vi "sendValveSignal-v02.2.vi"(0 "daq_do":tag="Dev1/ai0:1", 3 "Valve1?":bool, 5 "ChangeToValve":u16, 9 "CurrentValve":u16, 11 "controls array in":refnum<vi>[](array[refnum]), 12 "Set Status":bool, 13 "error in":errorcluster) -> (6 "ValveSetTo":u16, 10 "valve changed?":bool, 14 "error out":errorcluster, 15 "control array out":refnum<vi>[](array[refnum]))   [LabVIEW 2019]
uses:
  <vilib>/DAQmx/write.llb/DAQmx Write (Digital 1D Bool NChan 1Samp 1Line).vi
  <vilib>/DAQmx/miscellaneous.llb/DAQmx Fill In Error Info.vi
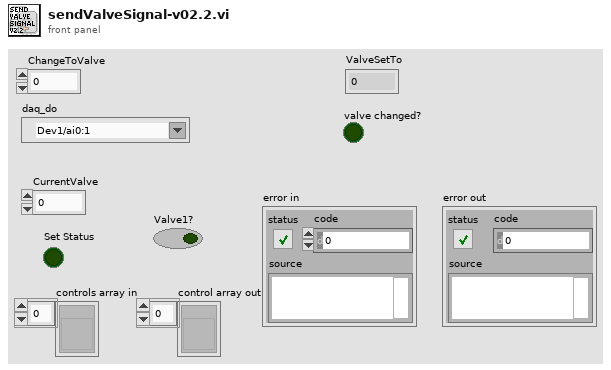
[diagram p1: front panel]
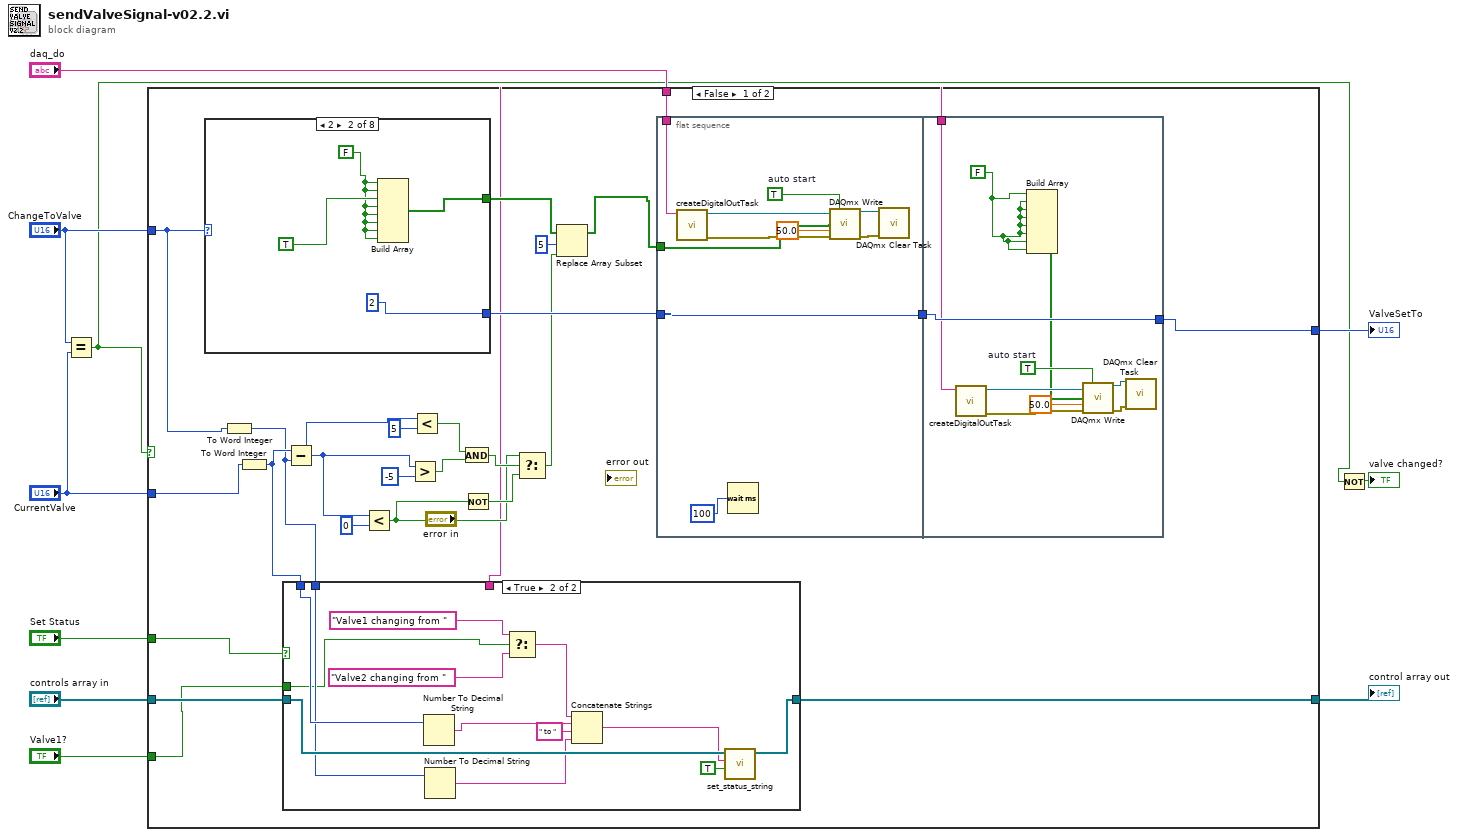
[diagram p0: block diagram]
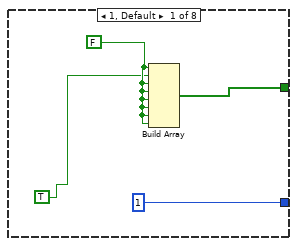
[diagram p3: hidden frame]
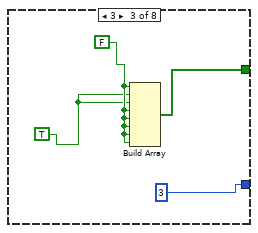
[diagram p4: hidden frame]
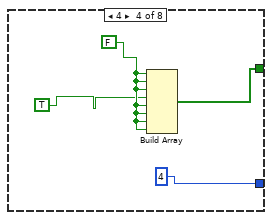
[diagram p5: hidden frame]
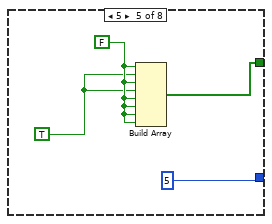
[diagram p6: hidden frame]
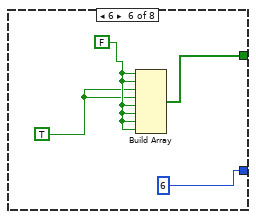
[diagram p7: hidden frame]
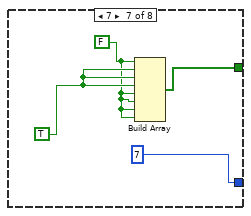
[diagram p8: hidden frame]
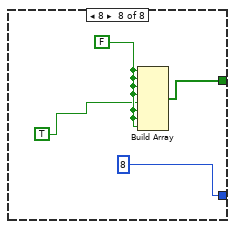
[diagram p9: hidden frame]
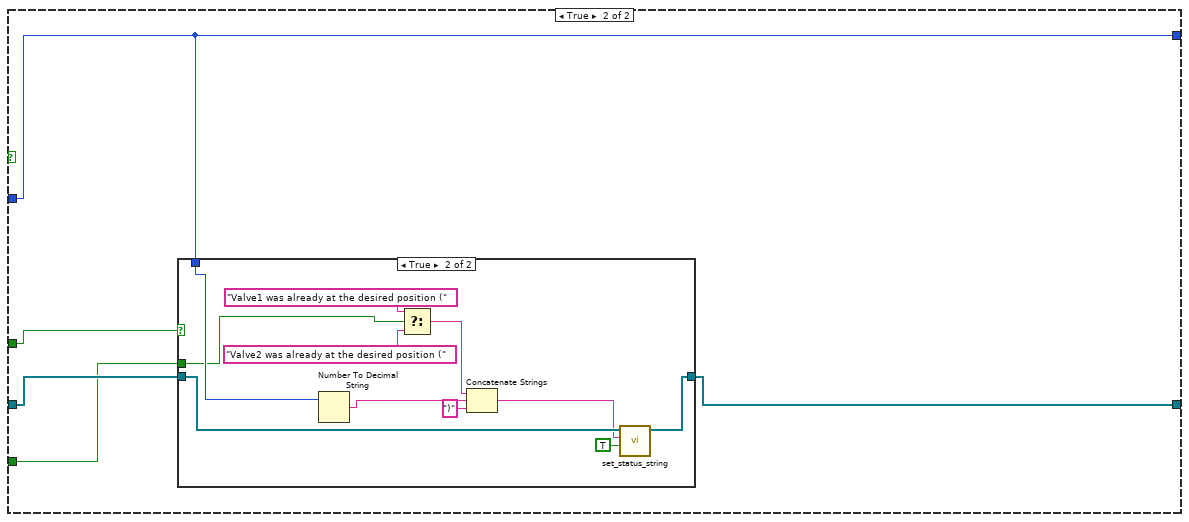
[diagram p10: hidden frame]
diagram:
  n1 = Equal?(x="ChangeToValve", y="CurrentValve") -> (x = y?=w1:bool)
  n2 = case shown="False" w1 {
    tunnel: [w33 w103] -> w10
    tunnel: "Set Status" -> [w19 w106]
    tunnel: "controls array in" -> [w18 w105]
    tunnel: [w17 w102] -> w7
    tunnel: "daq_do" -> [w16 _]
    tunnel: "Valve1?" -> [w13 w104]
    tunnel: "ChangeToValve" -> [w12 _]
    tunnel: "CurrentValve" -> [w11 w103]
    frame False {
      n3 = case shown="2" w12 {
        tunnel: [w73 w77 w81 w85 w89 w93 w97 w101] -> w23
        tunnel: [u16 1 u16 2 u16 3 u16 4 u16 5 u16 6 u16 7 u16 8] -> w34
        frame 1, Default {
          w71 = FALSE
          n4 = Build Array(w71, TRUE, w71, w71, w71, w71, w71, w71) -> (w73:bool[])
        }
        frame 2 {
          w74 = FALSE
          n5 = Build Array(w74, w74, TRUE, w74, w74, w74, w74, w74) -> (w77:bool[])
        }
        frame 3 {
          w79 = FALSE
          w78 = TRUE
          n6 = Build Array(w79, w78, w78, w79, w79, w79, w79, w79) -> (w81:bool[])
        }
        frame 4 {
          w83 = FALSE
          n7 = Build Array(w83, w83, w83, TRUE, w83, w83, w83, w83) -> (w85:bool[])
        }
        frame 5 {
          w87 = FALSE
          w86 = TRUE
          n8 = Build Array(w87, w86, w87, w86, w87, w87, w87, w87) -> (w89:bool[])
        }
        frame 6 {
          w91 = FALSE
          w90 = TRUE
          n9 = Build Array(w91, w91, w90, w90, w91, w91, w91, w91) -> (w93:bool[])
        }
        frame 7 {
          w94 = FALSE
          w95 = TRUE
          n10 = Build Array(w94, w95, w95, w95, w94, w94, w94, w94) -> (w97:bool[])
        }
        frame 8 {
          w99 = FALSE
          n11 = Build Array(w99, w99, w99, w99, TRUE, w99, w99, w99) -> (w101:bool[])
        }
      }
      n12 = To Word Integer(number=w12) -> (16bit integer=w14:i16)
      n13 = To Word Integer(number=w11) -> (16bit integer=w15:i16)
      n14 = case shown="True" w19 {
        tunnel: [w36 w47] -> w17
        tunnel: w18 -> [w36 w48]
        tunnel: w16 -> [_ _]
        tunnel: w15 -> [_ w43]
        tunnel: w14 -> [_ w40]
        tunnel: w13 -> [_ w37]
        frame False {
        }
        frame True {
          n15 = Number To Decimal String(number=w43) -> (decimal integer string=w42:string)  [unwired: 1 in]
          n16 = Number To Decimal String(number=w40) -> (decimal integer string=w39:string)  [unwired: 1 in]
          n17 = Select(t="Valve1 changing from ", s=w37, f="Valve2 changing from ") -> (s? t:f=w44:string)
          n18 = Concatenate Strings(w44, w42, " to " ("string"), w39) -> (w38:string)
          n19 = call "set_status_string.vi"("new line?"=TRUE, "status string in"=w38, "controls array"=w48) -> ("controls array out"=w47:refnum<vi>[])  [unwired: 7 in, 1 out]
        }
      }
      n20 = Subtract(x=w15, y=w14) -> (x-y=w30:i16)
      n21 = Less?(x=w30, y=i16 0) -> (x < y?=w24:bool)
      n22 = Greater?(x=w30, y=i16 -5) -> (0:w27:bool)
      n23 = Less?(x=w30, y=i16 5) -> (x < y?=w28:bool)
      n24 = And(x=w28, y=w27) -> (x .and. y?=w26:bool)
      n25 = Not(x=w24) -> (.not. x?=w25:bool)
      n26 = Select(t=w24, s=w26, f=w25) -> (s? t:f=w20:bool)
      n27 = Replace Array Subset(array=w23, new element=w20, index=5) -> (w22:bool[])
      n28 = flat-sequence {
        tunnel: w16 -> [w54]
        tunnel: w22 -> [w55]
        tunnel: w34 -> [w53]
        tunnel: [w53] -> w35
        tunnel: w35 -> [w69]
        tunnel: [w69] -> w33
        tunnel: w16 -> [w64]
        frame #0 {
          w58 = TRUE  # auto start
          n29 = call "createDigitalOutTask.vi"("daq_do"=w54) -> ("error out"=w56:errorcluster, "task out"=w57:refnum<k21>)  [unwired: 9 in]
          n30 = Wait (ms)(milliseconds to wait=u32 100) -> ()  [unwired: 1 out]
          n31 = call-poly <vilib>:"DAQmx Write.vi"("task/channels in"=w57, "auto start"=w58, "data"=w55, "timeout"=50.0, "error in"=w56) -> ("task out"=w51:refnum<k21>, "error out"=w50:errorcluster)  [unwired: 8 in, 1 out]
          n32 = call <vilib>:"DAQmx Clear Task.vi"("task in"=w51, "error in"=w50) -> ()  [unwired: 13 in, 1 out]
        }
        frame #1 {
          w62 = FALSE
          w68 = TRUE  # auto start
          n33 = call "createDigitalOutTask.vi"("daq_do"=w64) -> ("error out"=w66:errorcluster, "task out"=w67:refnum<k21>)  [unwired: 9 in]
          n34 = Build Array(w62, w62, w62, w62, w62, w62, w62, w62) -> (w65:bool[])
          n35 = call-poly <vilib>:"DAQmx Write.vi"("task/channels in"=w67, "auto start"=w68, "data"=w65, "timeout"=50.0, "error in"=w66) -> ("task out"=w61:refnum<k21>, "error out"=w60:errorcluster)  [unwired: 8 in, 1 out]
          n36 = call <vilib>:"DAQmx Clear Task.vi"("task in"=w61, "error in"=w60) -> ()  [unwired: 13 in, 1 out]
        }
      }
    }
    frame True {
      n37 = case shown="True" w106 {
        tunnel: [w107 w116] -> w102
        tunnel: w105 -> [w107 w117]
        tunnel: w103 -> [_ w112]
        tunnel: w104 -> [_ w108]
        frame False {
        }
        frame True {
          n38 = Number To Decimal String(number=w112) -> (decimal integer string=w111:string)  [unwired: 1 in]
          n39 = Select(t="Valve1 was already at the desired position (", s=w108, f="Valve2 was already at the desired position (") -> (s? t:f=w113:string)
          n40 = Concatenate Strings(w113, w111, ")" ("string")) -> (w109:string)
          n41 = call "set_status_string.vi"("new line?"=TRUE, "status string in"=w109, "controls array"=w117) -> ("controls array out"=w116:refnum<vi>[])  [unwired: 7 in, 1 out]
        }
      }
    }
  }
  "ValveSetTo" <- w10
  "control array out" <- w7
  n42 = Not(x=w1) -> (.not. x?=→"valve changed?":bool)
